vi "Main.vi"() -> ()   [LabVIEW 2018]
uses:
  FoodItem.ctl
  FEP.ctl
panel:
  out "Total Entries":i32 format="Total Entries: %.0f"
  out "size(s)":i32 format="Entries: %.0f"
  in  "Show":bool
  in  "Sausage show":u16(ring) caption="Sausage" items=["Badger Botillo", "Bear Salami", "Beaver Dog", "Big Bear Banger", "Boar Baloney", "Boar Boudin", "Butcher's Surprise", "Cavedog", "Chicken Chorizo", "Cow Chorizo", "Delicious Deer Dog", "Elk Dog", "Fox Fuet", "Fox Wurst", "Glazed Grazer Dog", "Hedgedog", "King of the Woods", "Lamb & Lynx", "Lamb Sausages", "Lynxalami", "Moodog", "Piglet Wursts", "Running Rabbit Sausage", "Swan Neck", "Tame Game Liverwurst", "Wonderful Wilderness Wurst"]
  in  "Stop":bool
  in  "Clear":bool
  out "Info":string[][](array[string])
  in  "Tree":u16(ring) caption="Smoked with" items=["RAW", "Alder", "Almond", "Apple", "Ash", "Aspen", "Bay Willow", "Beech", "Birch", "Birdcherry", "Black Pine", "Buckthorn", "Carob", "Cedar", "Chaste", "Cherry", "Chestnut", "Conker", "Cork Oak", "Crabapple", "Cypress", "Dogwood", "Elm", "Fir", "Gloomcap", "Gnome's Hat", "Goldenchain", "Hazel", "Hornbeam", "Juniper", "King's Oak", "Larch", "Laurel", "Lemon", "Linden", "Lote", "Maple", "Mayflower", "Medlar", "Mulberry", "Oak", "Olive", "Pear", "Persimmon", "Pine", "Plane", "Plum", "Poplar", "Quince", "Rowan", "Sallow", "Silver Fir", "Sorb", "Spruce", "Stone Pine", "Sweetgum", "Sycamore", "Terebinth", "Towercap", "Tree Heath", "Trumpet Chantrelle", "Walnut", "Whitebeam", "Willow", "Wood Strawberry", "Yew"]
  in  "Add":bool
  in  "Food":T1={"Q"=10.0, "Hunger"=0.0, "Energy"=0, "FEP"={"STR"={"+1"=0.0, "+2"=0.0}, "AGI"={"+1"=0.0, "+2"=0.0}, "INT"={"+1"=0.0, "+2"=0.0}, "CON"={"+1"=0.0, "+2"=0.0}, "PRC"={"+1"=0.0, "+2"=0.0}, "CHA"={"+1"=0.0, "+2"=0.0}, "DEX"={"+1"=0.0, "+2"=0.0}, "WIL"={"+1"=0.0, "+2"=0.0}, "PSY"={"+1"=0.0, "+2"=0.0}}} {"Q" format="%.1f"; "FEP"."PSY"."+2" format="%#.2f"; "FEP"."PSY"."+1" format="%#.2f"; "FEP"."WIL"."+2" format="%#.2f"; "FEP"."WIL"."+1" format="%#.2f"; "FEP"."DEX"."+2" format="%#.2f"; "FEP"."DEX"."+1" format="%#.2f"; "FEP"."CHA"."+2" format="%#.2f"; "FEP"."CHA"."+1" format="%#.2f"; "FEP"."PRC"."+2" format="%#.2f"; "FEP"."PRC"."+1" format="%#.2f"; "FEP"."CON"."+2" format="%#.2f"; "FEP"."CON"."+1" format="%#.2f"; "FEP"."INT"."+2" format="%#.2f"; "FEP"."INT"."+1" format="%#.2f"; "FEP"."AGI"."+2" format="%#.2f"; "FEP"."AGI"."+1" format="%#.2f"; "FEP"."STR"."+2" format="%#.2f"; "FEP"."STR"."+1" format="%#.2f"; "Energy" format="%.0f%"; "Hunger" format="%#.2f%"}
  in  "Sausage":u16(ring) items=["Badger Botillo", "Bear Salami", "Beaver Dog", "Big Bear Banger", "Boar Baloney", "Boar Boudin", "Butcher's Surprise", "Cavedog", "Chicken Chorizo", "Cow Chorizo", "Delicious Deer Dog", "Elk Dog", "Fox Fuet", "Fox Wurst", "Glazed Grazer Dog", "Hedgedog", "King of the Woods", "Lamb & Lynx", "Lamb Sausages", "Lynxalami", "Moodog", "Piglet Wursts", "Running Rabbit Sausage", "Swan Neck", "Tame Game Liverwurst", "Wonderful Wilderness Wurst"]
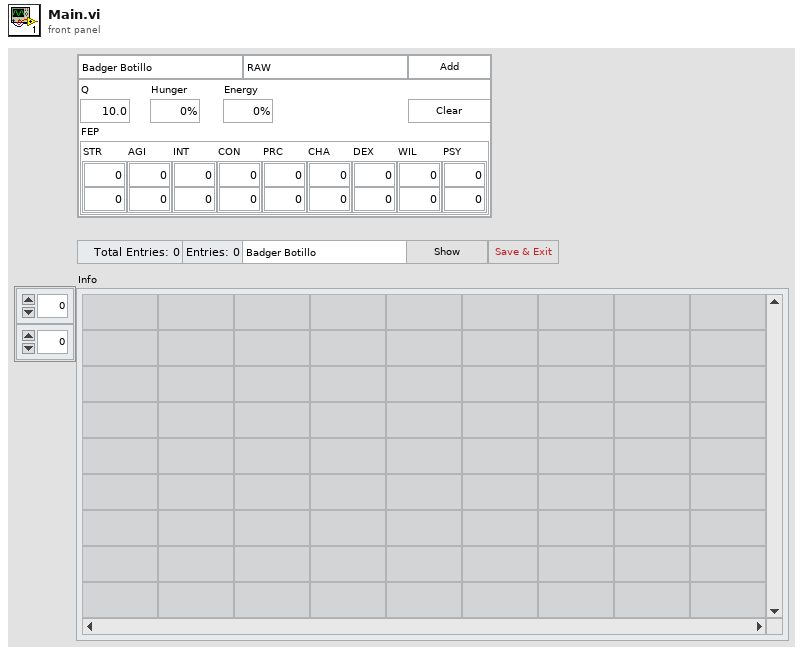
[diagram p1: front panel]
types:
  T1 = typedef "FoodItem.ctl" = cluster{"Q":dbl, "Hunger":dbl, "Energy":i32, "FEP":T2}
  T2 = typedef "FEP.ctl" = cluster{"STR":cluster{"+1":dbl, "+2":dbl}, "AGI":cluster{"+1":dbl, "+2":dbl}, "INT":cluster{"+1":dbl, "+2":dbl}, "CON":cluster{"+1":dbl, "+2":dbl}, "PRC":cluster{"+1":dbl, "+2":dbl}, "CHA":cluster{"+1":dbl, "+2":dbl}, "DEX":cluster{"+1":dbl, "+2":dbl}, "WIL":cluster{"+1":dbl, "+2":dbl}, "PSY":cluster{"+1":dbl, "+2":dbl}}
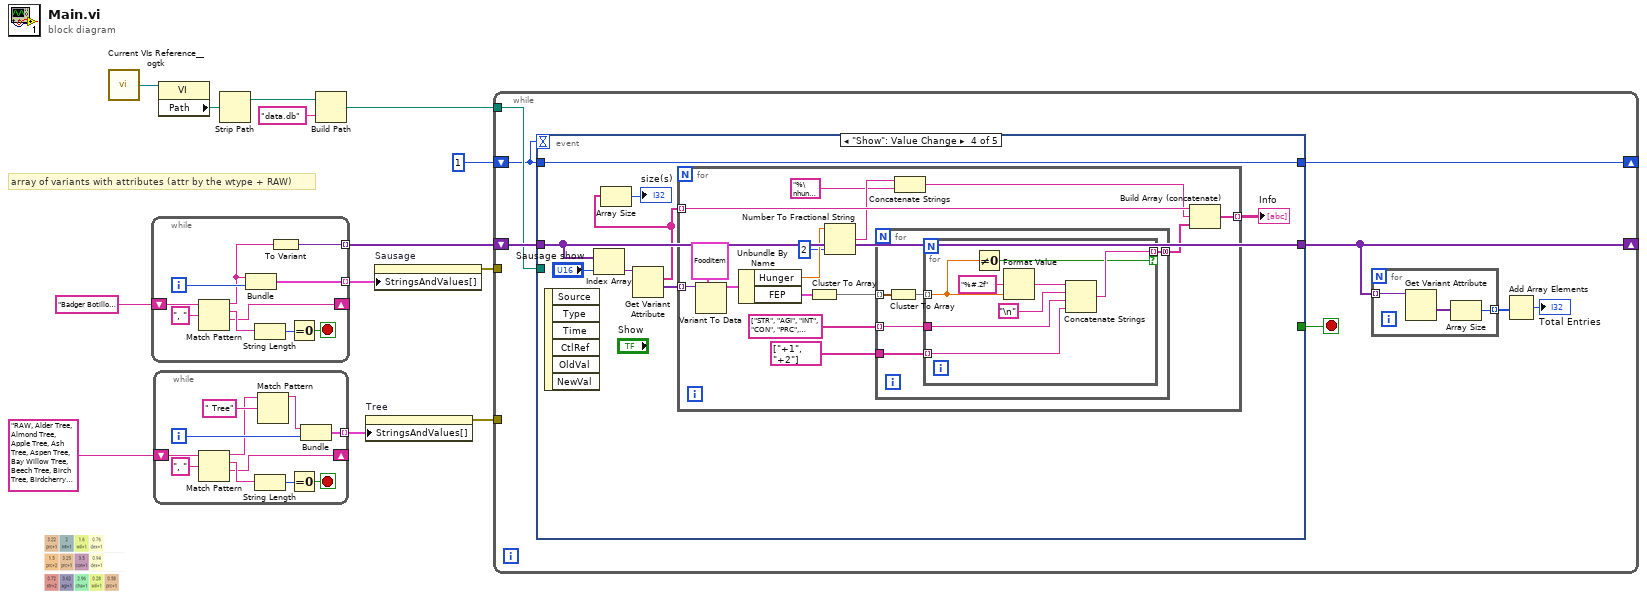
[diagram p0: block diagram]
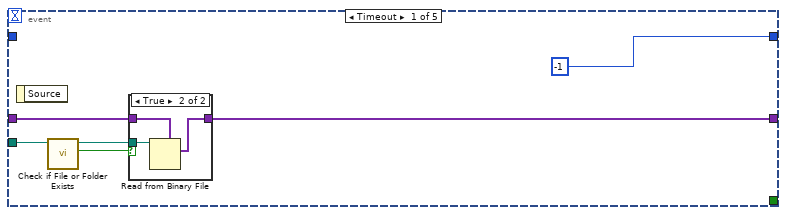
[diagram p2: hidden frame]
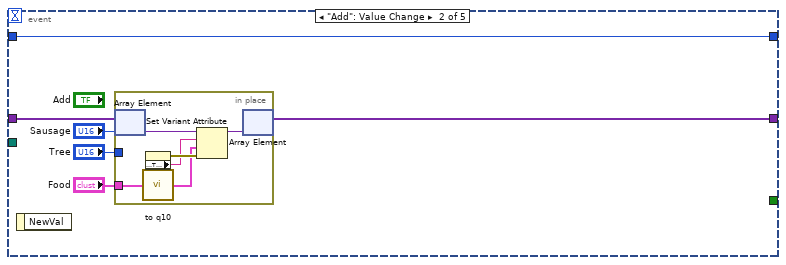
[diagram p4: hidden frame]
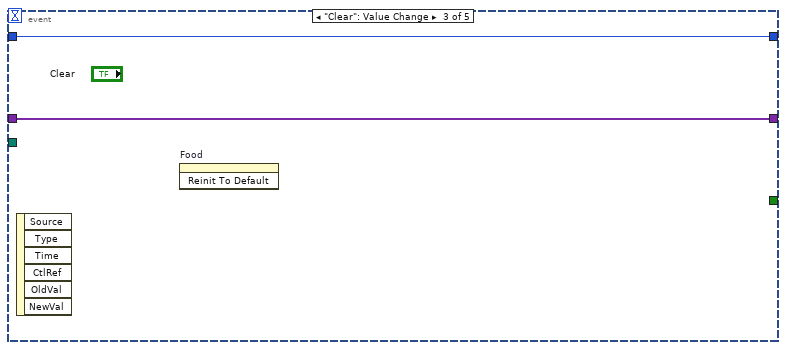
[diagram p5: hidden frame]
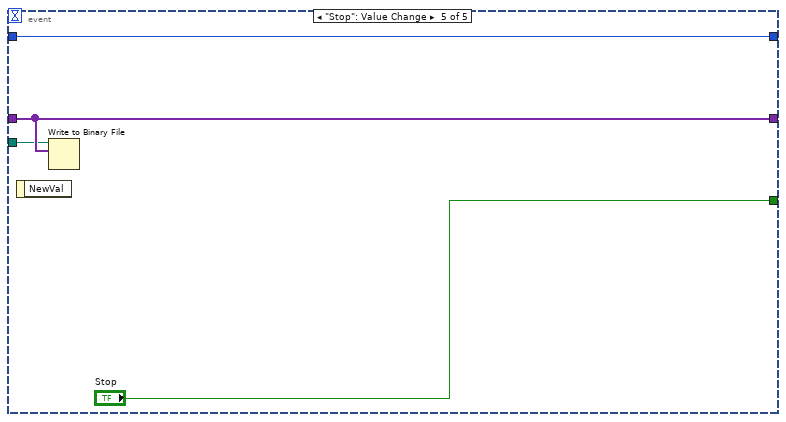
[diagram p6: hidden frame]
diagram:
  # "array of variants with attributes (attr by the wtype + RAW)"
  n1 = call <userlib>:"Current VIs Reference__ogtk.vi"() -> ("Current VI's reference"=w4:refnum<vi>)  [unwired: 5 in]
  n2 = while {
    shift-right: [w18] -> _
    shift-left: "Badger Botillo, Bear Salami, Beaver Dog, Big Bear Banger, Boar Baloney, Boar Boudin, Butcher's Surprise, Cavedog, Chicken Chorizo, Cow Chorizo, Delicious Deer Dog, Elk Dog, Fox Fuet, Fox Wurst, Glazed Grazer Dog, Hedgedog, King of the Woods, Lamb & Lynx, Lamb Sausages, Lynxalami, Moodog, Piglet Wursts, Running Rabbit Sausage, Swan Neck, Tame Game Liverwurst, Wonderful Wilderness Wurst" -> [w23]
    tunnel: [w16] -> w12 mode=indexing
    tunnel: [w14] -> w11 mode=indexing
    i -> [w17]
    stop <- w19 stop-if-true
    n3 = Match Pattern(string=w23, regular expression=", ") -> (before substring=w15:string, match substring=w21:string, after substring=w18:string)  [unwired: 1 in, 1 out]
    n4 = Bundle(w15, w17) -> (w16:cluster{string, i32})  [unwired: 1 in]
    n5 = String Length(string=w21) -> (length=w20:i32)
    n6 = To Variant(anything=w15) -> (Variant=w14:variant)
    n7 = Equal To 0?(x=w20) -> (x = 0?=w19:bool)
  }
  n8 = while {
    shift-right: [w27] -> _
    shift-left: "RAW, Alder Tree, Almond Tree, Apple Tree, Ash Tree, Aspen Tree, Bay Willow Tree, Beech Tree, Birch Tree, Birdcherry Tree, Black Pine Tree, Buckthorn Tree, Carob Tree, Cedar Tree, Chaste Tree, Cherry Tree, Chestnut Tree, Conker Tree, Cork Oak Tree, Crabapple Tree, Cypress Tree, Dogwood Tree, Elm Tree, Fir Tree, Gloomcap, Gnome's Hat, Goldenchain Tree, Hazel Tree, Hornbeam Tree, Juniper Tree, King's Oak Tree, Larch Tree, Laurel Tree, Lemon Tree, Linden Tree, Lote Tree, Maple Tree, Mayflower Tree, Medlar Tree, Mulberry Tree, Oak Tree, Olive Tree, Pear Tree, Persimmon Tree, Pine Tree, Plane Tree, Plum Tree, Poplar Tree, Quince Tree, Rowan Tree, Sallow Tree, Silver Fir Tree, Sorb Tree, Spruce Tree, Stone Pine Tree, Sweetgum Tree, Sycamore Tree, Terebinth Tree, Towercap, Tree Heath Tree, Trumpet Chantrelle, Walnut Tree, Whitebeam Tree, Willow Tree, Wood Strawberry Tree, Yew Tree" -> [w34]
    tunnel: [w28] -> w8 mode=indexing
    i -> [w29]
    stop <- w30 stop-if-true
    n9 = Match Pattern(string=w34, regular expression=", ") -> (before substring=w24:string, match substring=w32:string, after substring=w27:string)  [unwired: 1 in, 1 out]
    n10 = String Length(string=w32) -> (length=w31:i32)
    n11 = Match Pattern(string=w24, regular expression=" Tree") -> (before substring=w25:string)  [unwired: 1 in, 3 out]
    n12 = Equal To 0?(x=w31) -> (x = 0?=w30:bool)
    n13 = Bundle(w25, w29) -> (w28:cluster{string, i32})  [unwired: 1 in]
  }
  n14 = property class="VI"(reference=w4) -> ("Path"=w5:path)  [unwired: 1 in, 2 out]
  n15 = Strip Path(path=w5) -> (stripped path=w6:path)  [unwired: 1 out]
  n16 = Build Path(base path=w6, name or relative path="data.db") -> (appended path=w3:path)
  n17 = property on="Tree" class="Ring (strict)"("StringsAndValues[]"=w8) -> (error out=w9:errorcluster)  [unwired: 2 in, 1 out]
  n18 = property on="Sausage" class="Ring (strict)"("StringsAndValues[]"=w12) -> (error out=w7:errorcluster)  [unwired: 2 in, 1 out]
  n19 = while {
    shift-right: [w37] -> _
    shift-left: w11 -> [w41]
    tunnel: w9 -> [_]
    tunnel: w7 -> [_]
    tunnel: w3 -> [w40]
    shift-right: [w39] -> _
    shift-left: 1 -> [w38]
    stop <- w42 stop-if-true
    n20 = event shown="[3] \"Show\": Value Change" {
      selector: _ -> [_ _ _ _ _]
      dyn-events: _ -> [_ _ _ _ _]
      timeout: w38 -> [_ _ _ _ _]
      tunnel: [_ _ _ _ "Stop"] -> w42
      tunnel: w41 -> [w50 w61 w69 w76 w108]
      tunnel: [w51 w57 w69 w76 w108] -> w37
      tunnel: w40 -> [w47 _ _ _ w107]
      tunnel: [-1 w56 w68 w77 w106] -> w39
      tunnel: w38 -> [_ w56 w68 w77 w106]
      event Timeout {
        n21 = event-data() -> ()  [unwired: 1 in, 1 out]
        n22 = call <vilib>:"Check if File or Folder Exists.vi"("path"=w47) -> ("file or folder exists?"=w46:bool, "dup path"=w48:path)  [unwired: 8 in, 1 out]
        n23 = case shown="True" w46 {
          tunnel: [w52 w55] -> w51
          tunnel: w50 -> [w52 w54]
          tunnel: w48 -> [_ w53]
          frame False {
          }
          frame True {
            n24 = Read from Binary File(5:w54, 11:w53) -> (2:w55:variant[])  [unwired: 4 in, 3 out]
          }
        }
      }
      event "Add": Value Change {
        n25 = event-data() -> ()  [unwired: 1 in, 1 out]
        n26 = in-place {
          in-place-border: "Tree" -> [_]
          in-place-border: "Food" -> [w63]
          n27 = in-place-array #1(w61, "Sausage") -> (w66:variant)
          n28 = call "to q10.vi"("Food Item In"=w63) -> ("Food Item Out"=w62:T1)  [unwired: 6 in]
          n29 = property on="Tree" class="Ring (strict)"() -> (error out=w67:errorcluster, "RingText.Text"=w65:string)  [unwired: 2 in, 1 out]
          n30 = Set Variant Attribute(Variant=w66, name=w65, value=w62, error in=w67) -> (Variant out=w64:variant)  [unwired: 2 out]
          n31 = in-place-array #1(w64) -> (w57:variant[])  [unwired: 1 out]
        }
      }
      event "Clear": Value Change {
        n32 = event-data() -> ()  [unwired: 1 in, 6 out]
        n33 = invoke on="Food" class="Clust (strict)" method="Reinit To Default"() -> ()  [unwired: 3 in, 3 out]
      }
      event "Show": Value Change {
        n34 = event-data() -> ()  [unwired: 1 in, 6 out]
        n35 = Index Array(array=w76, index="Sausage show") -> (element=w74:variant)
        n36 = Get Variant Attribute(Variant=w74) -> (names=w71:string[], values=w73:variant[])  [unwired: 3 in, 2 out]
        n37 = Array Size(array=w71) -> (size(s)=→"size(s)":i32)
        n38 = for {
          tunnel: w73 -> [w92] mode=indexing
          tunnel: w71 -> [w81] mode=indexing
          tunnel: [w84] -> w72 mode=indexing
          n39 = Variant To Data(type=T1 {"Q"=121.5, "Hunger"=2.0, "Energy"=400, "FEP"={"STR"={"+1"=22.0, "+2"=0.0}, "AGI"={"+1"=2.0, "+2"=0.0}, "INT"={"+1"=0.0, "+2"=0.0}, "CON"={"+1"=0.0, "+2"=0.0}, "PRC"={"+1"=0.0, "+2"=0.0}, "CHA"={"+1"=0.0, "+2"=0.0}, "DEX"={"+1"=0.0, "+2"=0.0}, "WIL"={"+1"=0.0, "+2"=0.0}, "PSY"={"+1"=0.0, "+2"=0.0}}} ("Item"), Variant=w92) -> (data=w90:T1)  [unwired: 1 in, 1 out]
          n40 = Unbundle By Name(w90) -> ("Hunger"=w83:dbl, "FEP"=w89:T2)
          n41 = Cluster To Array(cluster=w89) -> (array=w88:cluster{"+1":dbl, "+2":dbl}[])
          n42 = Number To Fractional String(number=w83, precision (6)=i16 2) -> (F-format string=w80:string)  [unwired: 2 in]
          n43 = for {
            tunnel: w88 -> [w97] mode=indexing
            tunnel: string[] ["STR", "AGI", "INT", "CON", "PRC", "CHA", "DEX", "WIL", "PSY"] ("Text") -> [w94] mode=indexing
            tunnel: string[] ["+1", "+2"] ("Text") -> [w95]
            tunnel: [w93] -> w85 mode=concatenating
            n44 = Cluster To Array(cluster=w97) -> (array=w96:dbl[])
            n45 = for {
              tunnel: w96 -> [w105] mode=indexing
              tunnel: w95 -> [w103] mode=indexing
              tunnel: w94 -> [w104]
              tunnel: [w99] -> w93 mode=indexing if=w98
              n46 = Not Equal To 0?(x=w105) -> (x != 0?=w98:bool)
              n47 = Format Value(format string="%#.2f", value (0)=w105) -> (output string=w100:string)  [unwired: 1 in]
              n48 = Concatenate Strings(w100, "\n", w104, w103) -> (w99:string)
            }
          }
          n49 = Concatenate Strings(w80, "%\nhunger" ("string")) -> (w78:string)
          n50 = Build Array (concatenate)(w81, w78, w85) -> (w84:string[])
        }
        "Info" <- w72
      }
      event "Stop": Value Change {
        n51 = event-data() -> ()  [unwired: 1 in, 1 out]
        n52 = Write to Binary File(file (use dialog)=w107, data=w108) -> ()  [unwired: 4 in, 3 out]
      }
    }
    n53 = for {
      tunnel: w37 -> [w45] mode=indexing
      tunnel: [w43] -> w36 mode=indexing
      n54 = Get Variant Attribute(Variant=w45) -> (values=w44:variant[])  [unwired: 3 in, 3 out]
      n55 = Array Size(array=w44) -> (size(s)=w43:i32)
    }
    n56 = Add Array Elements(numeric array=w36) -> (sum=→"Total Entries":i32)
  }
